vi "CalculateMeanAndStDevForResultsInRange.vi"(11 "X":dbl[](array[numeric]) format="%0.2f") -> (1 "standard deviation":dbl format="%0.2f", 3 "mean":dbl format="%0.2f")   [LabVIEW 2013]
uses:
  <vilib>/Analysis/NI_AALBase.lvlib
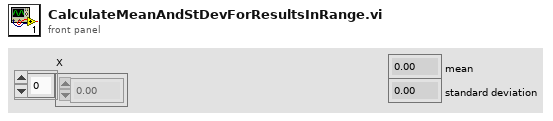
[diagram p1: front panel]
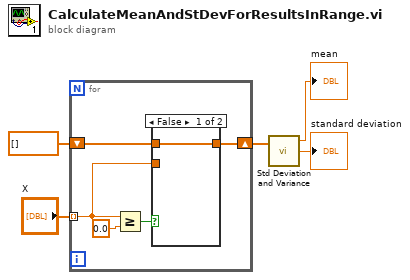
[diagram p0: block diagram]
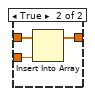
[diagram p2: hidden frame]
diagram:
  n1 = for {
    tunnel: "X" -> [w6] mode=indexing
    shift-right: [w9] -> w3
    shift-left: dbl[] [] ("array") -> [w10]
    n2 = Greater Or Equal?(x=w6, y=0.0) -> (x >= y?=w7:bool)
    n3 = case shown="False" w7 {
      tunnel: w10 -> [w11 w14]
      tunnel: [w11 w12] -> w9
      tunnel: w6 -> [_ w13]
      frame False {
      }
      frame True {
        n4 = Insert Into Array(array=w14, new element=w13) -> (w12:dbl[])  [unwired: 1 in]
      }
    }
  }
  n5 = call <vilib>:"Std Deviation and Variance.vi"("X"=w3) -> ("mean"=→"mean":dbl, "standard deviation"=→"standard deviation":dbl)  [unwired: 1 in, 1 out]
